vi "GetInstrumentsList.vi"(8 "error in (no error)":errorcluster, 11 "ByteGSWebAPI-V0 in":refnum<class "ByteGSWebAPI-V0.lvclass">) -> (0 "error out":errorcluster, 2 "InstrumentsList":T1, 3 "ByteGSWebAPI-V0 out":refnum<class "ByteGSWebAPI-V0.lvclass">)   [LabVIEW 2019, in "ByteGSWebAPI-V0.lvclass"]
doc: "Richiesta di GET di tutti gli strumenti (ID: \" \")"
uses:
  ByteGSWebAPI-V0.lvclass
  Cntrls/MultipleInstruments.ctl
  Cntrls/SingleInstrument.ctl
  cafd0801-0ee5-4417-b853-6a6d16c7dcb3.vi
  <vilib>/JDP Science/JSONtext/JSON text to Variant.vi
  <vilib>/JDP Science/JSONtext/LVClass Serializer/JSONtext LVClass Serializer.lvclass
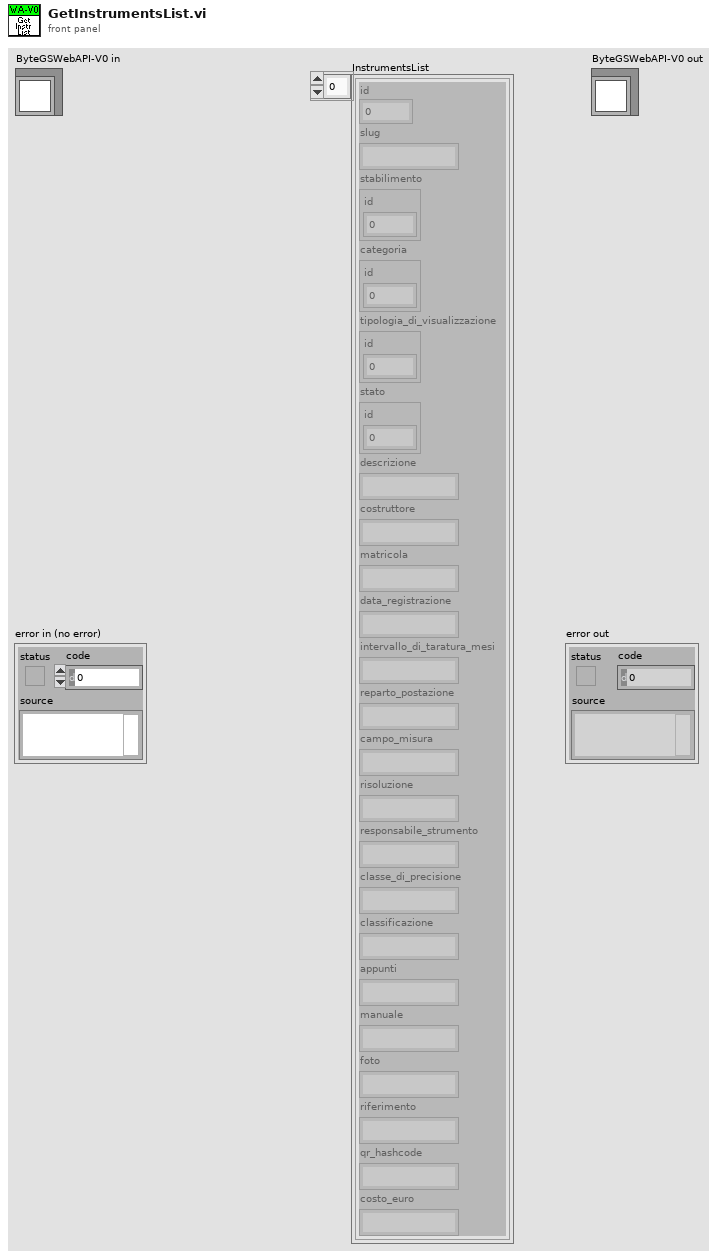
[diagram p1: front panel]
types:
  T1 = typedef "ByteGSWebAPI-V0.lvclass/MultipleInstruments.ctl" = T2[]
  T2 = typedef "ByteGSWebAPI-V0.lvclass/SingleInstrument.ctl" = cluster{"id":i32, "slug":string, "stabilimento":cluster{"id":dbl}, "categoria":cluster{"id":dbl}, "tipologia_di_visualizzazione":cluster{"id":dbl}, "stato":cluster{"id":dbl}, "descrizione":string, "costruttore":string, "matricola":string, "data_registrazione":string, "intervallo_di_taratura_mesi":string, "reparto_postazione":string, "campo_misura":string, "risoluzione":string, "responsabile_strumento":string, "classe_di_precisione":string, "classificazione":string, "appunti":string, "manuale":string, "foto":string, "riferimento":string, "qr_hashcode":string, "costo_euro":string}
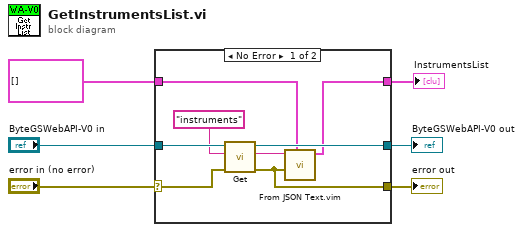
[diagram p0: block diagram]
diagram:
  n1 = case shown="No Error" "error in (no error)" {
    selector: "error in (no error)" -> [w12 w17]
    tunnel: [w7 w17] -> w5
    tunnel: [w11 w16] -> w3
    tunnel: "ByteGSWebAPI-V0 in" -> [w14 w16]
    tunnel: T1 [] ("MultipleInstruments") -> [w10 w15]
    tunnel: [w9 w15] -> w1
    frame No Error {
      n2 = call "Get.vi"("error in (no error)"=w12, "Request"="instruments" ("Parameter"), "ByteGSWebAPI-V0 in"=w14) -> ("error out"=w7:errorcluster, "body"=w8:string, "ByteGSWebAPI-V0 out"=w11:refnum<class "ByteGSWebAPI-V0.lvclass">)  [unwired: 5 in, 1 out]
      n3 = call "From JSON Text.vim"("Data Type and Default Value"=w10, "error in (no error)"=w7, "JSON"=w8) -> ("Data out"=w9:T1)  [unwired: 7 in, 1 out]
    }
    frame Error {
    }
  }
  "error out" <- w5
  "ByteGSWebAPI-V0 out" <- w3
  "InstrumentsList" <- w1
